vi "api_CheckConfig.vi"(8 "error in (no error)":errorcluster, 10 "needed_keys":string[](array[string]), 11 "ConfigClass_DVR":refnum<data-value>) -> (0 "error out":errorcluster, 1 "ok?":bool, 3 "ConfigClass_DVR_out":refnum<data-value>)   [LabVIEW 2019, in "ConfigClass.lvlib" / "ConfigClass.lvclass"]
uses:
  ConfigClass.lvclass
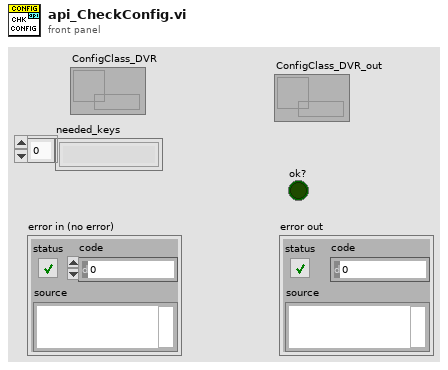
[diagram p1: front panel]
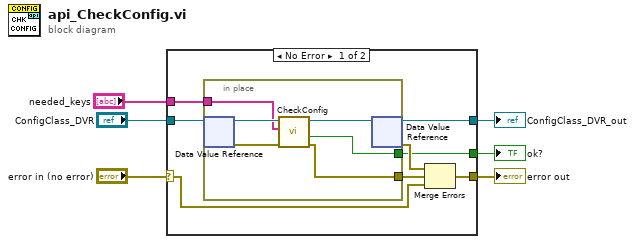
[diagram p0: block diagram]
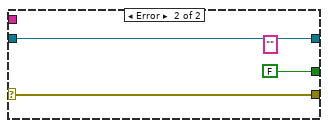
[diagram p2: hidden frame]
diagram:
  n1 = case shown="No Error" "error in (no error)" {
    selector: "error in (no error)" -> [w9 w23]
    tunnel: "ConfigClass_DVR" -> [w14 w22]
    tunnel: [w11 w23] -> w5
    tunnel: [w10 w22] -> w3
    tunnel: "needed_keys" -> [w8 _]
    tunnel: [w7 FALSE ("ok?")] -> w1
    frame No Error {
      n2 = in-place {
        in-place-border: [w16] -> w12
        in-place-border: w8 -> [w18]
        in-place-border: [w15] -> w7
        n3 = in-place-dvr #1(w14) -> (w20:refnum<class "ConfigClass.lvclass">, w17:errorcluster)
        n4 = call-dynamic "CheckConfig.vi"("error in (no error)"=w17, "needed_keys"=w18, "ConfigClass_IN"=w20) -> ("error out"=w16:errorcluster, "ok?"=w15:bool, "ConfigClass_OUT"=w19:refnum<class "ConfigClass.lvclass">)  [unwired: 6 in]
        n5 = in-place-dvr #1(w19) -> (w10:refnum<data-value>, w13:errorcluster)
      }
      n6 = Merge Errors(w13, w12, w9) -> (w11:errorcluster)
    }
    frame Error {
      (unwired) "" ("string_out")
    }
  }
  "ConfigClass_DVR_out" <- w3
  "error out" <- w5
  "ok?" <- w1
